vi "NanoStageGetMultPositions.vi"(7 "error in (no error)":errorcluster, 10 "Config In":T1 {"Hardware Configuration"."Lasers Configuration"."SettingValues"."785 Power" format="%.1f"; "Hardware Configuration"."Lasers Configuration"."SettingValues"."647 Power" format="%.1f"; "Hardware Configuration"."Lasers Configuration"."SettingValues"."561 Power" format="%.1f"; "Hardware Configuration"."Lasers Configuration"."SettingValues"."532 Power" format="%.1f"; "Hardware Configuration"."Lasers Configuration"."SettingValues"."488 Power" format="%.1f"; "Hardware Configuration"."Lasers Configuration"."SettingValues"."405 Power" format="%.1f"}) -> (0 "error out":errorcluster, 2 "Positions":cluster{"Time":dbl, "x":dbl, "y":dbl, "z":dbl}, 3 "Config Out":T1 {"Hardware Configuration"."Lasers Configuration"."SettingValues"."785 Power" format="%.1f"; "Hardware Configuration"."Lasers Configuration"."SettingValues"."647 Power" format="%.1f"; "Hardware Configuration"."Lasers Configuration"."SettingValues"."561 Power" format="%.1f"; "Hardware Configuration"."Lasers Configuration"."SettingValues"."532 Power" format="%.1f"; "Hardware Configuration"."Lasers Configuration"."SettingValues"."488 Power" format="%.1f"; "Hardware Configuration"."Lasers Configuration"."SettingValues"."405 Power" format="%.1f"})   [LabVIEW 2019]
doc: "Generates sample waveforms according to the signal type in the HW Config input."
uses:
  Settings/Settings.ctl
  Support/Hardware Configuration.ctl
  Support/Camera Configuration.ctl
  E:/DevHardSoftware/MMicroscopy/HardwareAdapter/Camera/Dependencies/PVCamNET.dll
  Camera/Dependencies/PVCamNET.dll
  <vilib>/userdefined/High Color/IMAQdx.ctl
  E:/DevHardSoftware/MMicroscopy/HardwareAdapter/Lasers/Dependencies/Oxxius_Boxx.dll
  Lasers/Dependencies/Oxxius_Boxx.dll
  Logging/Logging Configuration.ctl
  controls/UI Configuration.ctl
  <vilib>/numeric/Random Number (Range) U64.vi
  <vilib>/numeric/sub_Random U32.vi
  Global.vi
  Dependencies/Madlib.dll
  Logging/Logging.lvlib
  Settings/Settings.lvlib
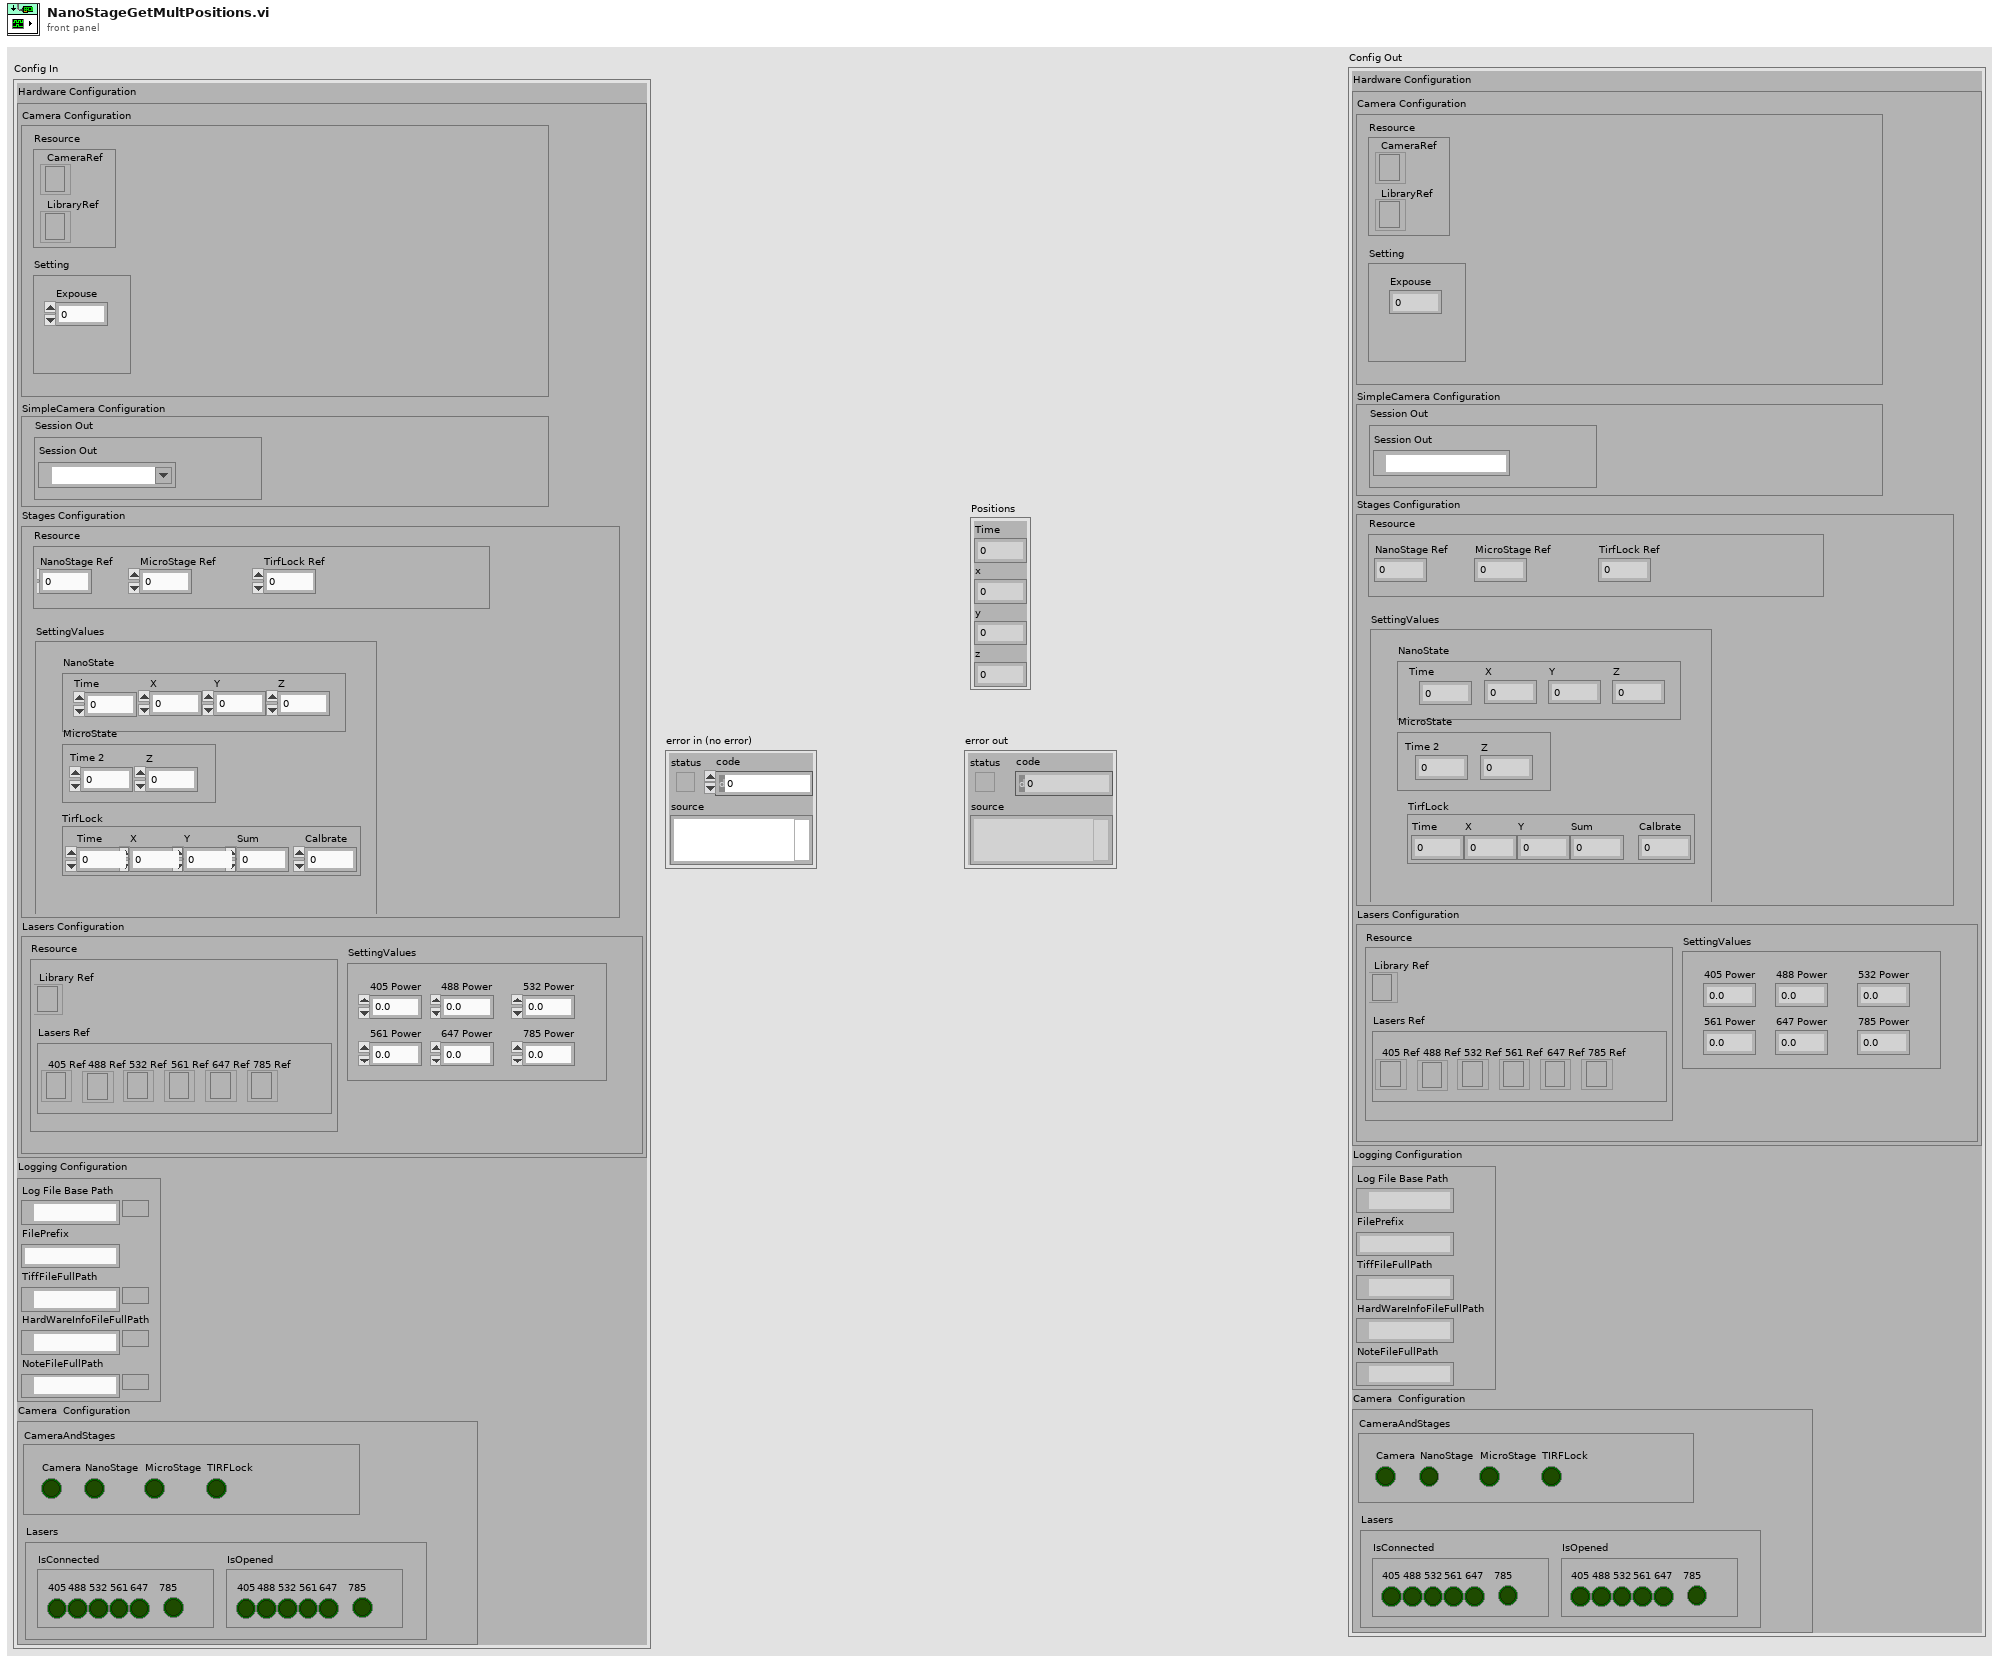
[diagram p1: front panel]
types:
  T1 = typedef "Settings.lvlib/Settings.ctl" = cluster{"Hardware Configuration":T2, "Logging Configuration":T5, "HardWare Status":cluster{"CameraAndStages":T6, "Lasers":cluster{"IsConnected":cluster{"405":bool, "488":bool, "532":bool, "561":bool, "647":bool, "785":bool}, "IsOpened":cluster{"405":bool, "488":bool, "532":bool, "561":bool, "647":bool, "785":bool}}}}
  T2 = typedef "Hardware Configuration.ctl" = cluster{"Camera Configuration":T3, "SimpleCamera Configuration":cluster{"Resource":cluster{"Session Out":T4}}, "Stages Configuration":cluster{"Resource":cluster{"NanoStage Ref":i32, "MicroStage Ref":i32, "TirfLock Ref":i32}, "SettingValues":cluster{"NanoState":cluster{"Time":dbl, "X":dbl, "Y":dbl, "Z":dbl}, "MicroState":cluster{"Time 2":dbl, "Z":dbl}, "TirfLock":cluster{"Time":dbl, "X":dbl, "Y":dbl, "Sum":dbl, "Calbrate":dbl}}}, "Lasers Configuration":cluster{"SettingValues":cluster{"405 Power":sgl, "488 Power":sgl, "532 Power":sgl, "561 Power":sgl, "647 Power":sgl, "785 Power":sgl}, "Resource":cluster{"Library Ref":refnum<k24>, "Lasers Ref":cluster{"405 Ref":refnum<k24>, "488 Ref":refnum<k24>, "532 Ref":refnum<k24>, "561 Ref":refnum<k24>, "647 Ref":refnum<k24>, "785 Ref":refnum<k24>}}}}
  T3 = typedef "Camera Configuration.ctl" = cluster{"Resource":cluster{"CameraRef":refnum<k24>, "LibraryRef":refnum<k24>}, "Setting":cluster{"Expouse":dbl}}
  T4 = typedef "IMAQdx.ctl" = refnum<k21>
  T5 = typedef "Logging.lvlib/Logging Configuration.ctl" = cluster{"Log File Base Path":path, "FilePrefix":string, "TiffFileFullPath":path, "HardWareInfoFileFullPath":path, "NoteFileFullPath":path}
  T6 = typedef "UI Configuration.ctl" = cluster{"Camera":bool, "NanoStage":bool, "MicroStage":bool, "TIRFLock":bool}
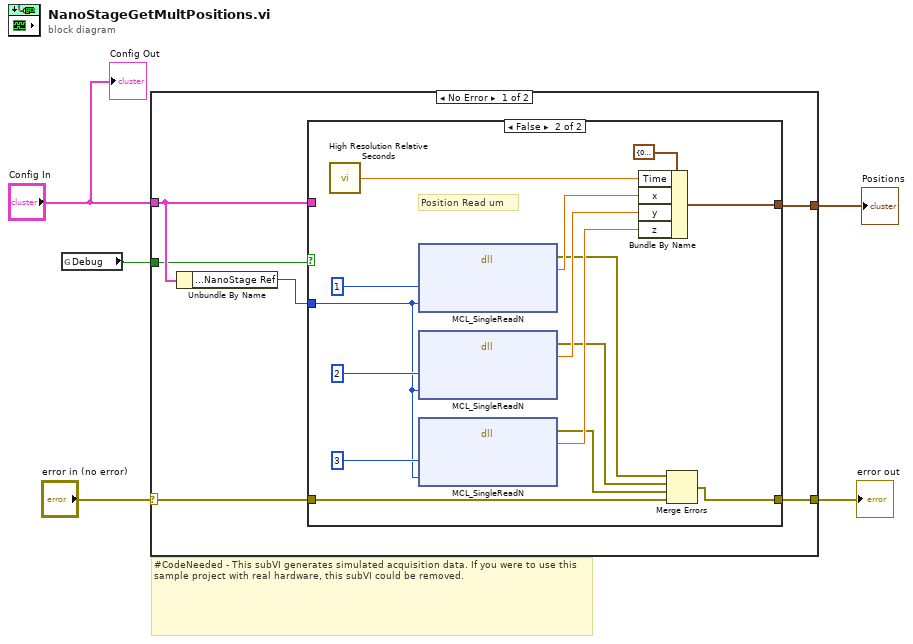
[diagram p0: block diagram]
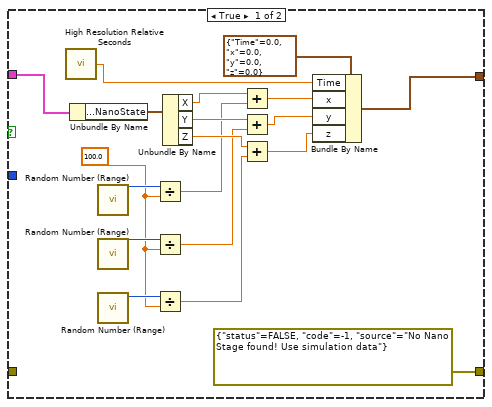
[diagram p2: hidden frame]
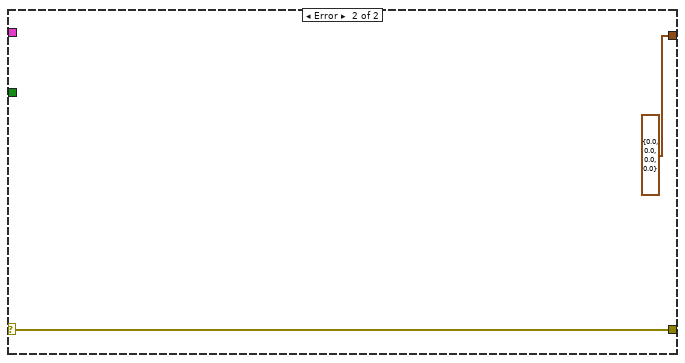
[diagram p3: hidden frame]
diagram:
  # "#CodeNeeded - This subVI generates simulated acquisition data. If you were to use this sample project with real hardware, this subVI could be removed."
  n1 = global read "Global.vi" "Debug"() -> (w1:bool)
  n2 = case shown="No Error" "error in (no error)" {
    selector: "error in (no error)" -> [w8 w46]
    tunnel: [w9 w46] -> w4
    tunnel: "Config In" -> [w7 _]
    tunnel: [w11 cluster{"Time":dbl, "x":dbl, "y":dbl, "z":dbl} {"Time"=0.0, "x"=0.0, "y"=0.0, "z"=0.0} ("RawImage")] -> w2
    tunnel: w1 -> [w6 _]
    frame No Error {
      n3 = Unbundle By Name(w7) -> ("Hardware Configuration.Stages Configuration.Resource.NanoStage Ref"=w10:i32)
      n4 = case shown="False" w6 {
        tunnel: [w28 w45] -> w11
        tunnel: w10 -> [_ w39]
        tunnel: [errorcluster {"status"=FALSE, "code"=-1, "source"="No Nano Stage found! Use simulation data"} ("error IO") w34] -> w9
        tunnel: w8 -> [_ w35]
        tunnel: w7 -> [w26 _]
        frame True {
          w15 = 100.0 ("Time")
          n5 = call <vilib>:"High Resolution Relative Seconds.vi"() -> ("relative seconds"=w27:dbl)
          n6 = Unbundle By Name(w26) -> ("Hardware Configuration.Stages Configuration.SettingValues.NanoState"=w25:cluster{"Time":dbl, "X":dbl, "Y":dbl, "Z":dbl})
          n7 = call-poly <vilib>:"Random Number (Range).vi"() -> ("number"=w24:u64)  [unwired: 11 in]
          n8 = call-poly <vilib>:"Random Number (Range).vi"() -> ("number"=w22:u64)  [unwired: 11 in]
          n9 = call-poly <vilib>:"Random Number (Range).vi"() -> ("number"=w23:u64)  [unwired: 11 in]
          n10 = Divide(x=w24, y=w15) -> (x/y=w16:dbl)
          n11 = Divide(x=w22, y=w15) -> (x/y=w17:dbl)
          n12 = Divide(x=w23, y=w15) -> (x/y=w18:dbl)
          n13 = Unbundle By Name(w25) -> ("X"=w21:dbl, "Y"=w20:dbl, "Z"=w19:dbl)
          n14 = Add(x=w21, y=w16) -> (x+y=w14:dbl)
          n15 = Add(x=w20, y=w17) -> (x+y=w13:dbl)
          n16 = Add(x=w19, y=w18) -> (x+y=w12:dbl)
          n17 = Bundle By Name(cluster=cluster{"Time":dbl, "x":dbl, "y":dbl, "z":dbl} {"Time"=0.0, "x"=0.0, "y"=0.0, "z"=0.0} ("NanoStage"), "Time"=w27, "x"=w14, "y"=w13, "z"=w12) -> (w28:cluster{"Time":dbl, "x":dbl, "y":dbl, "z":dbl})
        }
        frame False {
          # "Position Read um"
          n18 = call <vilib>:"High Resolution Relative Seconds.vi"() -> ("relative seconds"=w41:dbl)
          n19 = dll-call lib="E:/DevHardSoftware/MMicroscopy/HardwareAdapter/Stages/Dependencies/Madlib.dll" fn="MCL_SingleReadN"("axis"=u32 1, "handle"=w39) -> (error out=w31:errorcluster, w38:dbl)  [unwired: 5 in, 1 out]
          n20 = dll-call lib="E:/DevHardSoftware/MMicroscopy/HardwareAdapter/Stages/Dependencies/Madlib.dll" fn="MCL_SingleReadN"("axis"=u32 2, "handle"=w39) -> (error out=w32:errorcluster, w37:dbl)  [unwired: 5 in, 1 out]
          n21 = dll-call lib="E:/DevHardSoftware/MMicroscopy/HardwareAdapter/Stages/Dependencies/Madlib.dll" fn="MCL_SingleReadN"("axis"=u32 3, "handle"=w39) -> (error out=w33:errorcluster, w36:dbl)  [unwired: 5 in, 1 out]
          n22 = Bundle By Name(cluster=cluster{"Time":dbl, "x":dbl, "y":dbl, "z":dbl} {"Time"=0.0, "x"=0.0, "y"=0.0, "z"=0.0} ("RawImage"), "Time"=w41, "x"=w38, "y"=w37, "z"=w36) -> (w45:cluster{"Time":dbl, "x":dbl, "y":dbl, "z":dbl})
          n23 = Merge Errors(w31, w32, w33, w35) -> (w34:errorcluster)
        }
      }
    }
    frame Error {
    }
  }
  "error out" <- w4
  "Positions" <- w2
  "Config Out" <- "Config In"
